vi "call WCF library.vi"() -> ()   [LabVIEW 2013]
uses:
  System.ServiceModel
  G:/gitRepositories/TestProjects/WCFTest/WCFComputerLibrary/bin/Debug/WCFComputerLibrary.dll
  WCFComputerLibrary/bin/Debug/WCFComputerLibrary.dll
panel:
  out "StringToNumber":dbl
  out "Negate":dbl
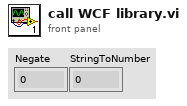
[diagram p1: front panel]
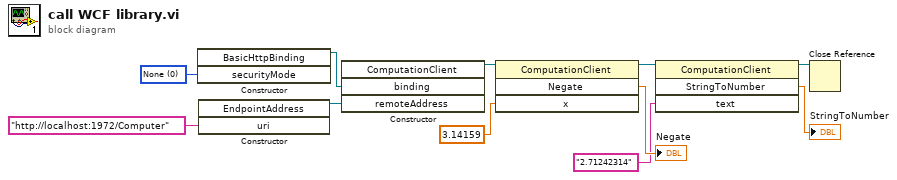
[diagram p0: block diagram]
diagram:
  w11 = 0 items=["None", "Transport", "Message", "TransportWithMessageCredential", "TransportCredentialOnly"] ("securityMode")
  n1 = constructor class="BasicHttpBinding"("securityMode"=w11) -> (reference out=w9:refnum<k24>)  [unwired: 3 in, 3 out]
  n2 = constructor class="EndpointAddress"("uri"="http://localhost:1972/Computer") -> (reference out=w8:refnum<k24>)  [unwired: 3 in, 3 out]
  n3 = constructor class="ComputationClient"("binding"=w9, "remoteAddress"=w8) -> (reference out=w7:refnum<k24>)  [unwired: 3 in, 4 out]
  n4 = invoke class="ComputationClient" method="Negate"(reference=w7, "x"=3.14159) -> (reference out=w4:refnum<k24>, "Negate"=→"Negate":dbl)  [unwired: 2 in, 2 out]
  n5 = invoke class="ComputationClient" method="StringToNumber"(reference=w4, "text"="2.71242314") -> (reference out=w1:refnum<k24>, "StringToNumber"=→"StringToNumber":dbl)  [unwired: 2 in, 2 out]
  n6 = Close Reference(reference=w1) -> ()  [unwired: 1 in, 1 out]
